vi "commongui_updateVariableList.vi"(8 "error in (no error)":errorcluster, 9 "Controls[]":refnum<vi>[](array[refnum]), 10 "Arguments":string, 11 "SQL Server Info":T2) -> (0 "error out":errorcluster)   [LabVIEW 2020]
uses:
  Shared/MySQL/typedefs/mysql_authentication.ctl
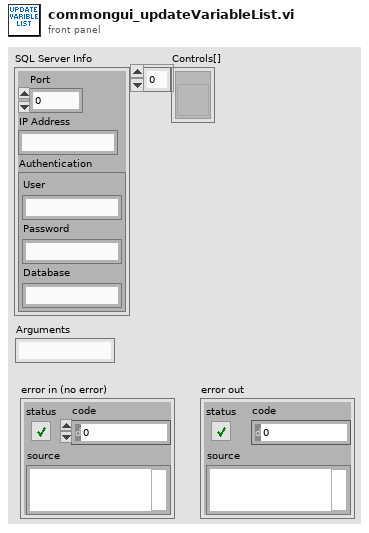
[diagram p1: front panel]
types:
  T1 = typedef "mysql_authentication.ctl" = cluster{"User":string, "Password":string, "Database":string}
  T2 = cluster{"Port":u16, "IP Address":string, "Authentication":T1}
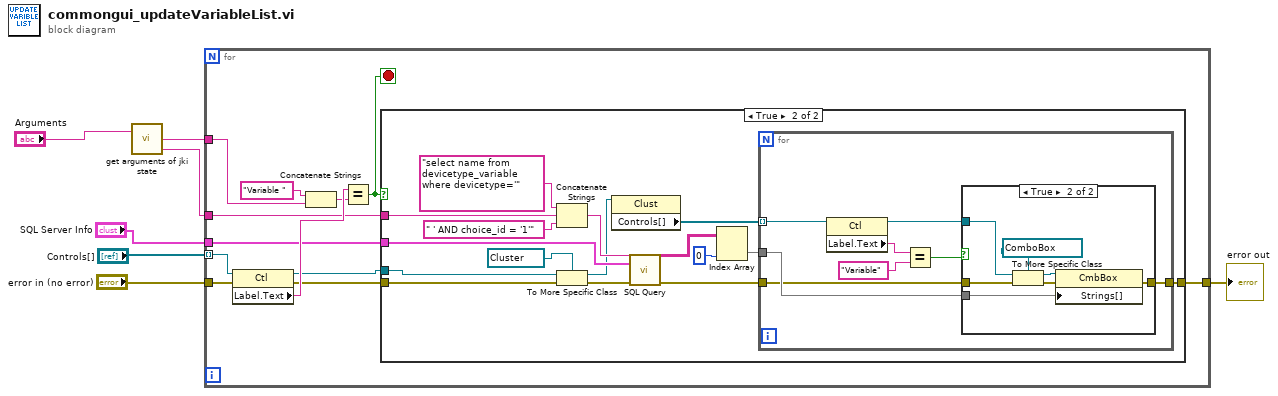
[diagram p0: block diagram]
diagram:
  n1 = call "get arguments of jki state.vi"("jki arguments"="Arguments") -> ("Arg 1"=w6:string, "Arg 2"=w7:string)  [unwired: 1 in, 1 out]
  n2 = for {
    tunnel: "Controls[]" -> [w19] mode=indexing
    tunnel: w6 -> [w10]
    tunnel: "error in (no error)" -> [w14]
    tunnel: "SQL Server Info" -> [w12]
    tunnel: [w11] -> w4
    tunnel: w7 -> [w9]
    stop <- w8 stop-if-true
    n3 = property class="Ctl"(reference=w19, error in=w14) -> (reference out=w16:refnum<vi>, error out=w15:errorcluster, "Label.Text"=w17:string)
    n4 = Concatenate Strings("Variable ", w10) -> (w13:string)
    n5 = Equal?(x=w17, y=w13) -> (x = y?=w8:bool)
    n6 = case shown="True" w8 {
      tunnel: w16 -> [_ w36]
      tunnel: w15 -> [w20 w35]
      tunnel: w9 -> [_ w29]
      tunnel: w12 -> [_ w27]
      tunnel: [w20 w24] -> w11
      frame False {
      }
      frame True {
        n7 = Concatenate Strings("select name from devicetype_variable where devicetype='" ("Query"), w29, " ' AND choice_id = '1'" ("string")) -> (w30:string)
        n8 = To More Specific Class(target class=refnum<vi> refnum ("Device 2"), reference=w36, error in=w35) -> (specific class reference=w22:refnum<vi>, error out=w26:errorcluster)
        n9 = property class="Clust"(reference=w22) -> ("Controls[]"=w21:refnum<vi>[])  [unwired: 1 in, 2 out]
        n10 = call "SQL Query.vi"("error in (no error)"=w26, "SQL Server Info"=w27, "Query"=w30) -> ("error out"=w25:errorcluster, "data"=w34:string[][])  [unwired: 7 in]
        n11 = Index Array(array=w34, index (col)=0 ("disabled index (col)")) -> (element=w28:string[])  [unwired: 1 in]
        n12 = for {
          tunnel: w28 -> [w44]
          tunnel: w25 -> [w42]
          tunnel: [w43] -> w24
          tunnel: w21 -> [w41] mode=indexing
          n13 = property class="Ctl"(reference=w41) -> (reference out=w38:refnum<vi>, "Label.Text"=w39:string)  [unwired: 1 in, 1 out]
          n14 = Equal?(x=w39, y="Variable") -> (x = y?=w37:bool)
          n15 = case shown="True" w37 {
            tunnel: w44 -> [_ w52]
            tunnel: [w45 w51] -> w43
            tunnel: w42 -> [w45 w48]
            tunnel: w38 -> [_ w46]
            frame False {
            }
            frame True {
              n16 = To More Specific Class(target class=refnum<vi> refnum ("Device 2"), reference=w46, error in=w48) -> (specific class reference=w49:refnum<vi>, error out=w47:errorcluster)
              n17 = property class="CmbBox"(reference=w49, error in=w47, "Strings[]"=w52) -> (error out=w51:errorcluster)  [unwired: 1 out]
            }
          }
        }
      }
    }
  }
  "error out" <- w4
